vi "Set Dev Margin.vi"(8 "error in (no error)":errorcluster, 9 "firmware revision":string(combo), 10 "dev margin (1.0)":dbl=1.0 min=1.0 max=20.0, 11 "VISA resource name":refnum<visa-resource-name>) -> (0 "error out":errorcluster, 2 "bridge error":T1, 3 "VISA resource name out":refnum<visa-resource-name>)   [LabVIEW 2020, in "Andeen-Hagerling 2700A.lvlib"]
doc: "Set the values of the deviation mode margin parameter.\n\nThe deviation margin which controls the ability of the\nbridge to handle deviations outside of the input deviation\nbounds without encountering overloading of the preamplidier."
uses:
  Andeen-Hagerling 2700A.lvlib
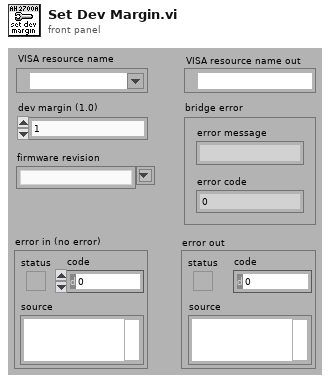
[diagram p1: front panel]
types:
  T1 = cluster{"error message":string, "error code":i32}
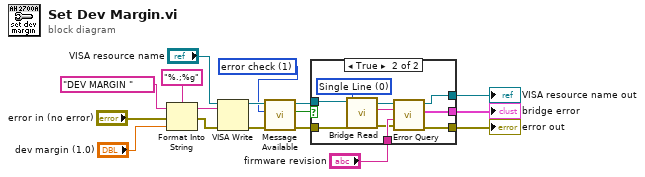
[diagram p0: block diagram]
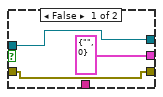
[diagram p2: hidden frame]
diagram:
  w1 = u16 1 items=["none", "error check", "multiline read", "infinite"] ("delay")
  n1 = Format Into String(format string="%.;%g", initial string="DEV MARGIN " ("command"), error in="error in (no error)", "dev margin (1.0)") -> (resulting string=w13:string, error out=w14:errorcluster)
  n2 = VISA Write(VISA resource name="VISA resource name", write buffer=w13, error in (no error)=w14) -> (VISA resource name out=w6:refnum<visa-resource-name>, error out=w5:errorcluster)  [unwired: 1 out]
  n3 = call "Message Available.vi"("error in (no error)"=w5, "delay"=w1, "VISA resource name"=w6) -> ("error out"=w8:errorcluster, "message available"=w10:bool, "VISA resource name out"=w9:refnum<visa-resource-name>)  [unwired: 6 in]
  n4 = case shown="True" w10 {
    tunnel: w9 -> [w19 w26]
    tunnel: w8 -> [w20 w25]
    tunnel: "firmware revision" -> [_ w30]
    tunnel: [w20 w29] -> w3
    tunnel: [w19 w28] -> w4
    tunnel: [T1 {"error message"="", "error code"=0} ("bridge error") w27] -> w2
    frame False {
    }
    frame True {
      w21 = u16 0 items=["Single Line", "Multi-Line"] ("Multiline")
      n5 = call "Bridge Read.vi"("error in (no error)"=w25, "multiline"=w21, "VISA resource name"=w26) -> ("error out"=w24:errorcluster, "read buffer"=w23:string, "VISA resource name out"=w22:refnum<visa-resource-name>)  [unwired: 6 in]
      n6 = call "Error Query.vi"("error in (no error)"=w24, "firmware revision"=w30, "measurement line"=w23, "VISA resource name"=w22) -> ("error out"=w29:errorcluster, "bridge error"=w27:T1, "VISA resource name out"=w28:refnum<visa-resource-name>)  [unwired: 5 in]
    }
  }
  "VISA resource name out" <- w4
  "error out" <- w3
  "bridge error" <- w2
